vi "SP_ZAction.vi"(8 "error in (no error)":errorcluster, 9 "Need Z?":bool, 10 "Z Action":T1(ring), 11 "SemiProbe in":refnum<class "SemiProbe.lvclass">) -> (0 "error out":errorcluster, 1 "previous Z [µm]":i32, 2 "Z [µm]":i32, 3 "SemiProbe out":refnum<class "SemiProbe.lvclass">)   [LabVIEW 2019, in "SemiProbe.lvclass"]
uses:
  SemiProbe.lvclass
  InstrumentSetup.vi
  <vilib>/Utility/error.llb/Error Cluster From Error Code.vi
  <vilib>/ErrorRing/Error Ring.xnode
  ArduinoControl/ArduinoControl.lvclass
  InstrControl.lvclass
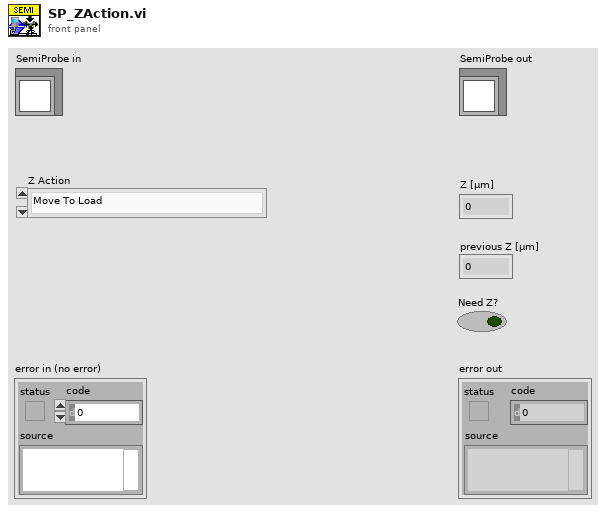
[diagram p1: front panel]
types:
  T1 = enum16{"Move To Load", "Move To Double Separation", "Move To Separation Distance", "Move To Contact", "Execute Contact Search", "Execute Arduino Contact Search"}
  T2 = cluster{"SP Load Less Than Thr?":bool, "SP Load Threshold (um)":dbl, "SP Current Location":cluster{"X (um)":ext, "Y (um)":ext, "Z (um)":ext, "T (degree)":ext}, "SP Chuck Speeds":cluster{"XY Speed (10-100%)":dbl, "Z Speed (10-100%)":dbl, "T Speed (10-100%)":dbl}, "Manual Step Parameters":cluster{"Step in X":bool, "X S-Speed [µm/step]":sgl, "Step in Y":bool, "Y S-Speed [µm/step]":sgl, "Step in Z":bool, "Z S-Speed [µm/step]":sgl, "Step in T":bool, "T S-Speed [mdegree/step]":sgl, "X Increase":bool, "Y Increase?":bool, "Z Increase?":bool, "T Increase?":bool}, "Z Stepper":cluster{"UP/DOWN":bool, "UP/DOWN Speed [µm/step]":i32, "SP Z Step":bool}, "Z Heights Set":bool, "SP Contact Search":cluster{"Contact Circuit":enum16{"12", "1", "2"}, "Speed [1000-10000]":sgl, "Start Height [µm]":sgl, "Search Band [µm]":sgl, "Overdrive [µm]":sgl}, "Separation Distance [µm]":u32, "Contact Height [µm]":u32, "Use Overdrive?":bool, "Touchdown method":enum16{"no feedback", "Arduino edgesense", "SP contact circuit"}, "Arduino Edgesense params":cluster{"touchdown height [µm]":i32, "search band [µm]":u32, "speed [µm/step]":u32, "overdrive [µm]":u32}}
  T3 = cluster{"Contact Circuit":enum16{"12", "1", "2"}, "Speed [1000-10000]":sgl, "Start Height [µm]":sgl, "Search Band [µm]":sgl, "Overdrive [µm]":sgl}
  T4 = cluster{"touchdown height [µm]":i32, "search band [µm]":u32, "speed [µm/step]":u32, "overdrive [µm]":u32}
  T5 = cluster{"VISA address":refnum<visa-resource-name>, "T sensor":enum16{"SHT", "DS"}, "Arduino":refnum<class "ArduinoControl.lvclass">}
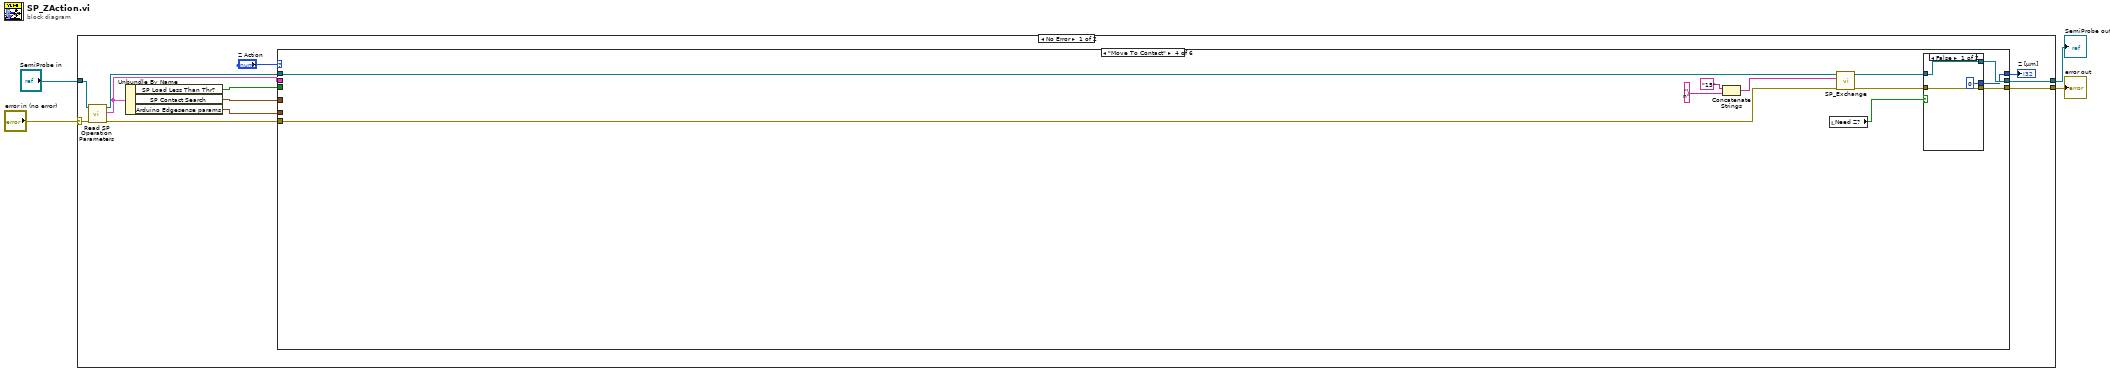
[diagram p0: block diagram]
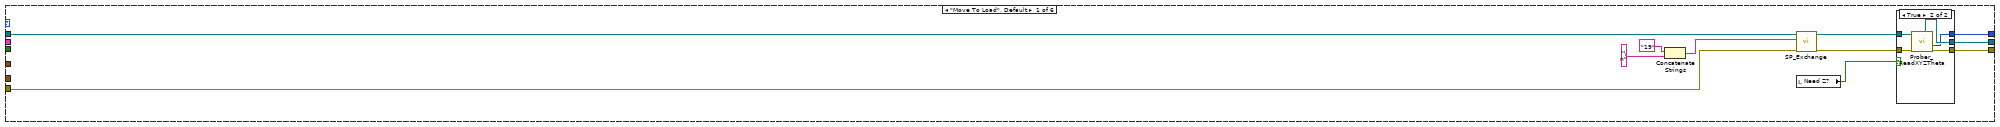
[diagram p2: hidden frame]
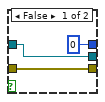
[diagram p3: hidden frame]
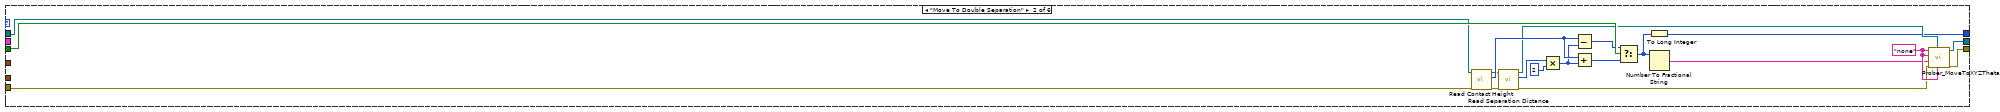
[diagram p4: hidden frame]
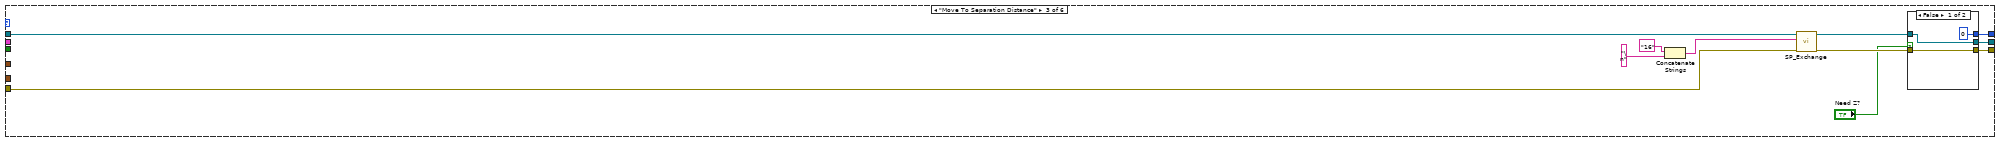
[diagram p5: hidden frame]
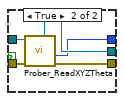
[diagram p6: hidden frame]
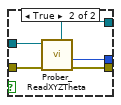
[diagram p7: hidden frame]
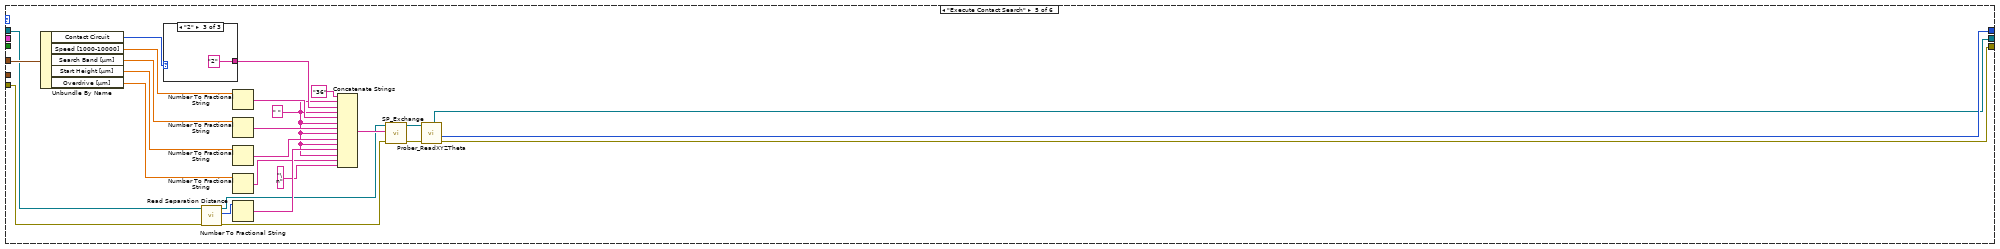
[diagram p8: hidden frame]
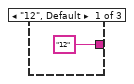
[diagram p9: hidden frame]
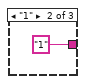
[diagram p10: hidden frame]
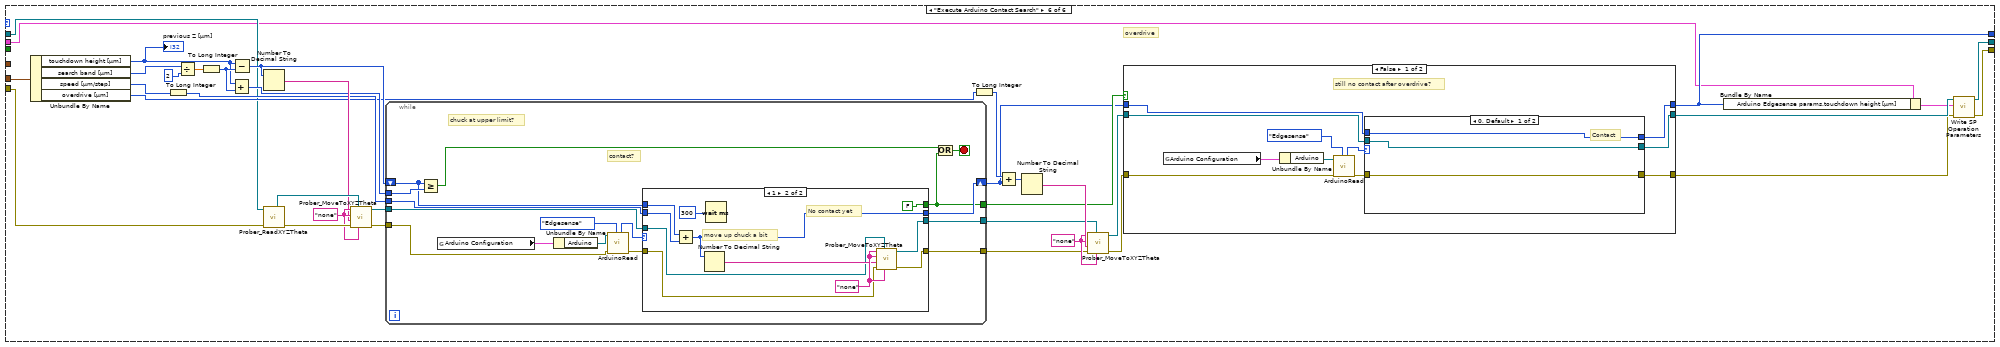
[diagram p11: hidden frame]
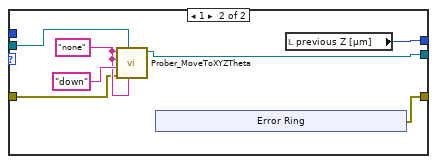
[diagram p12: hidden frame]
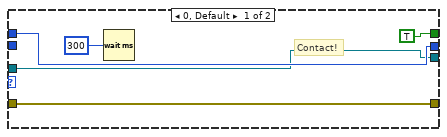
[diagram p14: hidden frame]
diagram:
  n1 = case shown="No Error" "error in (no error)" {
    selector: "error in (no error)" -> [w9 w220]
    tunnel: [w14 w220] -> w3
    tunnel: [w15 w219] -> w1
    tunnel: "SemiProbe in" -> [w13 w219]
    frame No Error {
      n2 = call-dynamic "Read SP Operation Parameters.vi"("error in (no error)"=w9, "SemiProbe in"=w13) -> ("error out"=w10:errorcluster, "SP Operation Parameters"=w5:T2, "SemiProbe out"=w11:refnum<class "SemiProbe.lvclass">)  [unwired: 7 in]
      n3 = Unbundle By Name(w5) -> ("SP Load Less Than Thr?"=w12:bool, "SP Contact Search"=w8:T3, "Arduino Edgesense params"=w6:T4)
      n4 = case shown="\"Move To Contact\"" "Z Action" {
        tunnel: [w21 w38 w60 w76 w96 w126] -> w15
        tunnel: [w22 w39 w57 w77 w98 w125] -> w14
        tunnel: w12 -> [_ w51 _ _ _ _]
        tunnel: w11 -> [w18 w44 w62 w81 w107 w130]
        tunnel: w10 -> [w19 w43 w61 w80 w106 w131]
        tunnel: w8 -> [_ _ _ _ w116 _]
        tunnel: [w20 w36 w56 w75 w97 w128] -> w7
        tunnel: w6 -> [_ _ _ _ _ w129]
        tunnel: w5 -> [_ _ _ _ _ w123]
        frame "Move To Load", Default {
          n5 = Concatenate Strings("19", "\n") -> (w25:string)
          n6 = call-dynamic "SP_Exchange.vi"("error in (no error)"=w19, "command"=w25, "SemiProbe in"=w18) -> ("error out"=w23:errorcluster, "SemiProbe out"=w24:refnum<class "SemiProbe.lvclass">)  [unwired: 4 in, 3 out]
          n7 = local read "Need Z?"() -> (w17:bool)
          n8 = case shown="True" w17 {
            tunnel: w24 -> [w30 w35]
            tunnel: w23 -> [w29 w34]
            tunnel: [w29 w33] -> w22
            tunnel: [w30 w32] -> w21
            tunnel: [0 ("Z location [µm]") w31] -> w20
            frame False {
            }
            frame True {
              n9 = call-dynamic "Prober_ReadXYZTheta.vi"("error in (no error)"=w34, "SemiProbe in"=w35) -> ("error out"=w33:errorcluster, "Z location [µm]"=w31:i32, "SemiProbe out"=w32:refnum<class "SemiProbe.lvclass">)  [unwired: 4 in, 3 out]
            }
          }
        }
        frame "Move To Double Separation" {
          w54 = "none"
          n10 = call-dynamic "Read Contact Height.vi"("error in (no error)"=w43, "SemiProbe in"=w44) -> ("error out"=w45:errorcluster, "Contact Height [µm]"=w48:u32, "SemiProbe out"=w46:refnum<class "SemiProbe.lvclass">)  [unwired: 7 in]
          n11 = call-dynamic "Read Separation Distance.vi"("error in (no error)"=w45, "SemiProbe in"=w46) -> ("error out"=w42:errorcluster, "Separation Distance"=w52:u32, "SemiProbe out"=w40:refnum<class "SemiProbe.lvclass">)  [unwired: 7 in]
          n12 = Multiply(x=w52, y=2) -> (x*y=w47:u32)
          n13 = Subtract(x=w48, y=w47) -> (x-y=w50:u32)
          n14 = Add(x=w48, y=w47) -> (x+y=w49:u32)
          n15 = Select(t=w50, s=w51, f=w49) -> (s? t:f=w37:u32)
          n16 = To Long Integer(number=w37) -> (32bit integer=w36:i32)
          n17 = Number To Fractional String(number=w37) -> (F-format string=w41:string)  [unwired: 3 in]
          n18 = call-dynamic "Prober_MoveToXYZTheta.vi"("Theta location [mdeg]"=w54, "SemiProbe in"=w40, "error in (no error)"=w42, "Z location [µm]"=w41, "Y location [µm]"=w54, "X location [µm]"=w54) -> ("error out"=w39:errorcluster, "SemiProbe out"=w38:refnum<class "SemiProbe.lvclass">)  [unwired: 3 in, 1 out]
        }
        frame "Move To Separation Distance" {
          n19 = Concatenate Strings("16", "\n") -> (w63:string)
          n20 = call-dynamic "SP_Exchange.vi"("error in (no error)"=w61, "command"=w63, "SemiProbe in"=w62) -> ("error out"=w58:errorcluster, "SemiProbe out"=w59:refnum<class "SemiProbe.lvclass">)  [unwired: 4 in, 3 out]
          n21 = case shown="False" "Need Z?" {
            tunnel: [w68 w73] -> w60
            tunnel: w59 -> [w68 w72]
            tunnel: w58 -> [w66 w71]
            tunnel: [w66 w70] -> w57
            tunnel: [0 ("Z location [µm]") w69] -> w56
            frame False {
            }
            frame True {
              n22 = call-dynamic "Prober_ReadXYZTheta.vi"("error in (no error)"=w71, "SemiProbe in"=w72) -> ("error out"=w70:errorcluster, "Z location [µm]"=w69:i32, "SemiProbe out"=w73:refnum<class "SemiProbe.lvclass">)  [unwired: 4 in, 3 out]
            }
          }
        }
        frame "Move To Contact" {
          n23 = Concatenate Strings("15", "\n") -> (w82:string)
          n24 = local read "Need Z?"() -> (w74:bool)
          n25 = call-dynamic "SP_Exchange.vi"("error in (no error)"=w80, "command"=w82, "SemiProbe in"=w81) -> ("error out"=w78:errorcluster, "SemiProbe out"=w79:refnum<class "SemiProbe.lvclass">)  [unwired: 4 in, 3 out]
          n26 = case shown="False" w74 {
            tunnel: w79 -> [w87 w92]
            tunnel: w78 -> [w86 w91]
            tunnel: [w86 w90] -> w77
            tunnel: [w87 w89] -> w76
            tunnel: [0 ("Z location [µm]") w88] -> w75
            frame False {
            }
            frame True {
              n27 = call-dynamic "Prober_ReadXYZTheta.vi"("error in (no error)"=w91, "SemiProbe in"=w92) -> ("error out"=w90:errorcluster, "Z location [µm]"=w88:i32, "SemiProbe out"=w89:refnum<class "SemiProbe.lvclass">)  [unwired: 4 in, 3 out]
            }
          }
        }
        frame "Execute Contact Search" {
          w101 = " "
          n28 = Unbundle By Name(w116) -> ("Contact Circuit"=w115:enum16{"12", "1", "2"}, "Speed [1000-10000]"=w113:sgl, "Search Band [µm]"=w112:sgl, "Start Height [µm]"=w111:sgl, "Overdrive [µm]"=w95:sgl)
          n29 = case shown="\"2\"" w115 {
            tunnel: ["12" "1" "2"] -> w114
            frame "12", Default {
            }
            frame "1" {
            }
            frame "2" {
            }
          }
          n30 = call-dynamic "Read Separation Distance.vi"("error in (no error)"=w106, "SemiProbe in"=w107) -> ("error out"=w94:errorcluster, "Separation Distance"=w105:u32, "SemiProbe out"=w93:refnum<class "SemiProbe.lvclass">)  [unwired: 7 in]
          n31 = Number To Fractional String(number=w113) -> (F-format string=w110:string)  [unwired: 3 in]
          n32 = Number To Fractional String(number=w112) -> (F-format string=w109:string)  [unwired: 3 in]
          n33 = Number To Fractional String(number=w111) -> (F-format string=w108:string)  [unwired: 3 in]
          n34 = Number To Fractional String(number=w95) -> (F-format string=w103:string)  [unwired: 3 in]
          n35 = Number To Fractional String(number=w105) -> (F-format string=w104:string)  [unwired: 3 in]
          n36 = Concatenate Strings("36", w101, w114, w101, w110, w101, w109, w101, w108, w101, w104, w101, w103, "\n") -> (w117:string)
          n37 = call-dynamic "SP_Exchange.vi"("error in (no error)"=w94, "command"=w117, "SemiProbe in"=w93) -> ("error out"=w99:errorcluster, "SemiProbe out"=w100:refnum<class "SemiProbe.lvclass">)  [unwired: 4 in, 3 out]
          n38 = call-dynamic "Prober_ReadXYZTheta.vi"("error in (no error)"=w99, "SemiProbe in"=w100) -> ("error out"=w98:errorcluster, "Z location [µm]"=w97:i32, "SemiProbe out"=w96:refnum<class "SemiProbe.lvclass">)  [unwired: 4 in, 3 out]
        }
        frame "Execute Arduino Contact Search" {
          w139 = "none" ("Z location")
          w150 = "none" ("Z location")
          # "overdrive"
          n39 = Unbundle By Name(w129) -> ("touchdown height [µm]"=w132:i32, "search band [µm]"=w156:u32, "speed [µm/step]"=w157:u32, "overdrive [µm]"=w143:u32)
          "previous Z [µm]" <- w132
          n40 = To Long Integer(number=w157) -> (32bit integer=w144:i32)
          n41 = Divide(x=w156, y=u32 2) -> (x/y=w154:dbl)
          n42 = To Long Integer(number=w154) -> (32bit integer=w153:i32)
          n43 = Add(x=w132, y=w153) -> (x+y=w148:i32)
          n44 = Subtract(x=w132, y=w153) -> (x-y=w147:i32)
          n45 = Number To Decimal String(number=w147) -> (decimal integer string=w149:string)  [unwired: 1 in]
          n46 = call-dynamic "Prober_ReadXYZTheta.vi"("error in (no error)"=w131, "SemiProbe in"=w130) -> ("error out"=w151:errorcluster, "SemiProbe out"=w152:refnum<class "SemiProbe.lvclass">)  [unwired: 4 in, 4 out]
          n47 = call-dynamic "Prober_MoveToXYZTheta.vi"("Theta location [mdeg]"=w150, "SemiProbe in"=w152, "error in (no error)"=w151, "Z location [µm]"=w149, "Y location [µm]"=w150, "X location [µm]"=w150) -> ("error out"=w146:errorcluster, "SemiProbe out"=w145:refnum<class "SemiProbe.lvclass">)  [unwired: 3 in, 1 out]
          n48 = while {
            tunnel: w148 -> [w197]
            shift-right: [w190] -> w133
            shift-left: w147 -> [w193]
            tunnel: w146 -> [w199]
            tunnel: w145 -> [w198]
            tunnel: w144 -> [w191]
            tunnel: [w189] -> w136
            tunnel: [w188] -> w138
            tunnel: [w187] -> w137
            stop <- w195 stop-if-true
            # "chuck at upper limit?"
            # "contact?"
            n49 = Greater Or Equal?(x=w193, y=w197) -> (x >= y?=w196:bool)
            n50 = global read "InstrumentSetup.vi" "Arduino Configuration"() -> (w202:T5)
            n51 = Unbundle By Name(w202) -> ("Arduino"=w201:refnum<class "ArduinoControl.lvclass">)
            n52 = call "ArduinoRead.vi"("Arduino function"=enum16{"T/RH", "Interlock", "Edgesense"}."Edgesense", "error in (no error)"=w199, "ArduinoControl in"=w201) -> ("error out"=w192:errorcluster, "Edgesense Status"=w194:u16)  [unwired: 3 in, 4 out]
            n53 = case shown="1" w194 {
              tunnel: w191 -> [_ w218]
              tunnel: w193 -> [w204 w209]
              tunnel: [w204 w208] -> w190
              tunnel: [TRUE FALSE] -> w189
              tunnel: w192 -> [w206 w214]
              tunnel: [w206 w213] -> w188
              tunnel: w198 -> [w203 w211]
              tunnel: [w203 w210] -> w187
              frame 0, Default {
                # "Contact!"
                n54 = Wait (ms)(milliseconds to wait=300) -> ()  [unwired: 1 out]
              }
              frame 1 {
                w216 = "none" ("Z location")
                # "No contact yet"
                # "move up chuck a bit"
                n55 = Add(x=w209, y=w218) -> (x+y=w208:i32)
                n56 = Number To Decimal String(number=w208) -> (decimal integer string=w215:string)  [unwired: 1 in]
                n57 = Wait (ms)(milliseconds to wait=300) -> ()  [unwired: 1 out]
                n58 = call-dynamic "Prober_MoveToXYZTheta.vi"("Theta location [mdeg]"=w216, "SemiProbe in"=w211, "error in (no error)"=w214, "Z location [µm]"=w215, "Y location [µm]"=w216, "X location [µm]"=w216) -> ("error out"=w213:errorcluster, "SemiProbe out"=w210:refnum<class "SemiProbe.lvclass">)  [unwired: 3 in, 1 out]
              }
            }
            n59 = Or(x=w196, y=w189) -> (x .or. y?=w195:bool)
          }
          n60 = To Long Integer(number=w143) -> (32bit integer=w142:i32)
          n61 = Add(x=w142, y=w133) -> (x+y=w141:i32)
          n62 = Number To Decimal String(number=w141) -> (decimal integer string=w140:string)  [unwired: 1 in]
          n63 = call-dynamic "Prober_MoveToXYZTheta.vi"("Theta location [mdeg]"=w139, "SemiProbe in"=w137, "error in (no error)"=w138, "Z location [µm]"=w140, "Y location [µm]"=w139, "X location [µm]"=w139) -> ("error out"=w134:errorcluster, "SemiProbe out"=w135:refnum<class "SemiProbe.lvclass">)  [unwired: 3 in, 1 out]
          n64 = case shown="False" w136 {
            tunnel: w135 -> [w162 w184]
            tunnel: w134 -> [w166 w185]
            tunnel: w133 -> [w161 w186]
            tunnel: [w160 w185] -> w124
            tunnel: [w159 w186] -> w128
            tunnel: [w158 w184] -> w127
            frame False {
              # "still no contact after overdrive?"
              n65 = global read "InstrumentSetup.vi" "Arduino Configuration"() -> (w168:T5)
              n66 = Unbundle By Name(w168) -> ("Arduino"=w167:refnum<class "ArduinoControl.lvclass">)
              n67 = call "ArduinoRead.vi"("Arduino function"=enum16{"T/RH", "Interlock", "Edgesense"}."Edgesense", "error in (no error)"=w166, "ArduinoControl in"=w167) -> ("error out"=w164:errorcluster, "Edgesense Status"=w163:u16)  [unwired: 3 in, 4 out]
              n68 = case shown="0, Default" w163 {
                tunnel: w164 -> [w170 w176]
                tunnel: w162 -> [w171 w175]
                tunnel: w161 -> [w169 _]
                tunnel: [w170 w174] -> w160
                tunnel: [w169 w173] -> w159
                tunnel: [w171 w172] -> w158
                frame 0, Default {
                  # "Contact"
                }
                frame 1 {
                  w177 = "none" ("Z location")
                  n69 = call-dynamic "Prober_MoveToXYZTheta.vi"("Theta location [mdeg]"=w177, "SemiProbe in"=w175, "error in (no error)"=w176, "Z location [µm]"="down", "Y location [µm]"=w177, "X location [µm]"=w177) -> ("SemiProbe out"=w172:refnum<class "SemiProbe.lvclass">)  [unwired: 3 in, 2 out]
                  n70 = xnode "Error Ring"() -> ("error out"=w174:errorcluster)
                  n71 = local read "previous Z [µm]"() -> (w173:i32)
                }
              }
            }
            frame True {
            }
          }
          n72 = Bundle By Name(cluster=w123, "Arduino Edgesense params.touchdown height [µm]"=w128) -> (w122:T2)
          n73 = call-dynamic "Write SP Operation Parameters.vi"("error in (no error)"=w124, "SP Operation Parameters"=w122, "SemiProbe in"=w127) -> ("error out"=w125:errorcluster, "SemiProbe out"=w126:refnum<class "SemiProbe.lvclass">)  [unwired: 7 in]
        }
      }
      "Z [µm]" <- w7
    }
    frame Error {
    }
  }
  "error out" <- w3
  "SemiProbe out" <- w1
